vi "Send Dialog Return Msg.vi"(8 "error in (no error)":errorcluster, 11 "Dialog Return Msg":refnum<class "Dialog Return Msg.lvclass">) -> (0 "error out":errorcluster)   [LabVIEW 2017, in "IDialogBox.lvlib" / "Dialog Return Msg.lvclass"]
doc: "<License>\nCopyright © 2017 Composed Systems, LLC | All rights reserved\nwww.composed.io\n\nAuthor: Ethan Stern <ethan.stern@composed.io>\n\nThis software is provided \"AS IS\" WITHOUT WARRANTIES, either express or implied, AND IS FOR EDUCATIONAL PURPOSES ONLY.\n</License>"
uses:
  Dialog Return Msg.lvclass
  C:/Git/mva-framework/Framework/AbstractMessages/PreAddressedMsg/PreAddressedMsg.lvclass
  <vilib>/ActorFramework/Message Enqueuer/Message Enqueuer.lvclass
  AbstractMessages/PreAddressedMsg/PreAddressedMsg.lvclass/PreAddressedMsg.ctl
  Dialog Return Msg.lvclass/Dialog Return Msg.ctl
  <vilib>/ActorFramework/Message Enqueuer/Message Enqueuer.lvclass/Message Enqueuer.ctl
  <vilib>/ActorFramework/Message Priority Queue/Priority Enqueue.vi
  AbstractMessages/PreAddressedMsg/PreAddressedMsg.lvclass
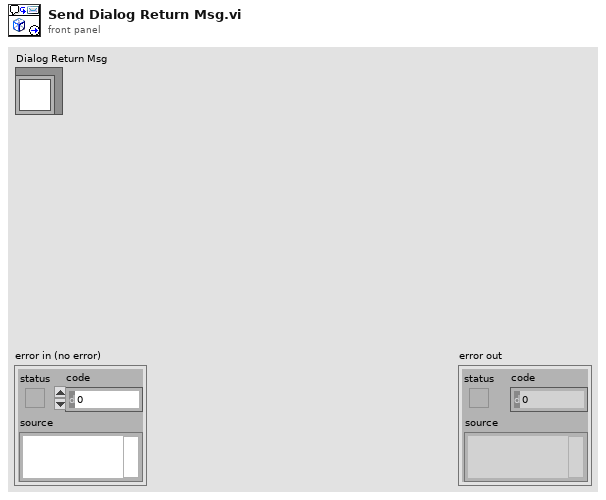
[diagram p1: front panel]
types:
  T1 = typedef "Actor Framework.lvlib/Message Enqueuer.lvclass/Message Priority.ctl" = enum16{"Low", "Normal", "High"}
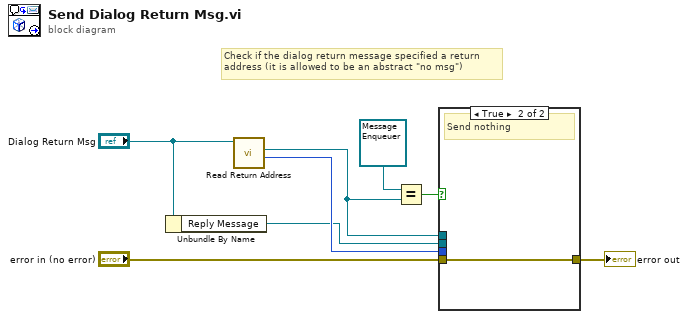
[diagram p0: block diagram]
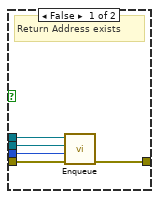
[diagram p2: hidden frame]
diagram:
  # "Check if the dialog return message specified a return\naddress (it is allowed to be an abstract \"no msg\")"
  n1 = Unbundle By Name("Dialog Return Msg") -> ("Reply Message"=w5:refnum<class "Message.lvclass">)
  n2 = call "Read Return Address.vi"("PreAddressedMsg in"="Dialog Return Msg") -> ("Return Priority (Normal)"=w7:T1, "Return Address"=w3:refnum<class "Message Enqueuer.lvclass">)  [unwired: 9 in]
  n3 = Equal?(x=refnum<class "Message Enqueuer.lvclass"> refnum ("Return Address"), y=w3) -> (x = y?=w1:bool)
  n4 = case shown="True" w1 {
    tunnel: "error in (no error)" -> [w13 w14]
    tunnel: w3 -> [w12 _]
    tunnel: w7 -> [w11 _]
    tunnel: w5 -> [w10 _]
    tunnel: [w9 w14] -> w4
    frame False {
      # "Return Address exists"
      n5 = call <vilib>:"Enqueue.vi"("error in (no error)"=w13, "Message Priority (Normal)"=w11, "Message"=w10, "Message Enqueuer in"=w12) -> ("error out"=w9:errorcluster)  [unwired: 6 in, 1 out]
    }
    frame True {
      # "Send nothing"
    }
  }
  "error out" <- w4
